vi "Init.vi"(7 "Options":T1, 8 "error in (no error)":errorcluster, 10 "Daemonized":bool, 11 "Execution in":refnum<class "Execution.lvclass">) -> (0 "error out":errorcluster, 3 "Execution out":refnum<class "Execution.lvclass">)   [LabVIEW 2020, in "TSnax.lvlib" / "Execution.lvclass"]
uses:
  Execution.lvclass
  Execution.lvclass/Execution.ctl
  Step Results.ctl
  Execution Options.ctl
  TSnax.lvlib
  Report/Report.lvclass
  SequenceFile/SequenceFile.lvclass
  PropertyObject/PropertyObject.lvclass
  Ref Data.ctl
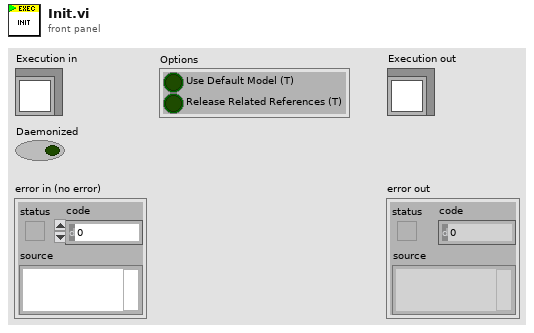
[diagram p1: front panel]
types:
  T1 = typedef "TSnax.lvlib/Execution Options.ctl" = cluster{"Use Default Model (T)":bool, "Release Related References (T)":bool}
  T2 = typedef "TSnax.lvlib/Execution.lvclass/Ref Data.ctl" = cluster{"Parameters":refnum<class "PropertyObject.lvclass">, "Client Sequence":refnum<class "SequenceFile.lvclass">, "Process Model":refnum<class "SequenceFile.lvclass">, "Entry Sequence":string, "Execution":refnum<k7>, "Report":refnum<class "Report.lvclass">, "Options":T1, "Started":bool, "Complete":bool}
  T3 = typedef "TSnax.lvlib/Execution.lvclass/Step Results.ctl" = cluster{"Map":map{string, string}}
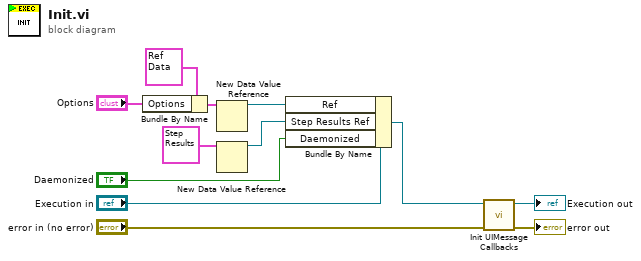
[diagram p0: block diagram]
diagram:
  n1 = Bundle By Name(cluster=T2 {"Parameters"=refnum, "Client Sequence"=refnum, "Process Model"=refnum, "Entry Sequence"="", "Execution"=refnum, "Report"=refnum, "Options"={"Use Default Model (T)"=FALSE, "Release Related References (T)"=FALSE}, "Started"=FALSE, "Complete"=FALSE} ("Ref Data"), "Options"="Options") -> (w9:T2)
  n2 = New Data Value Reference(data value=w9) -> (data value reference=w8:refnum<data-value>)  [unwired: 1 in, 1 out]
  n3 = New Data Value Reference(data value=T3 {"Map"={}} ("Step Results")) -> (data value reference=w6:refnum<data-value>)  [unwired: 1 in, 1 out]
  n4 = Bundle By Name(cluster="Execution in", "Ref"=w8, "Step Results Ref"=w6, "Daemonized"="Daemonized") -> (w3:refnum<class "Execution.lvclass">)
  n5 = call "Init UIMessage Callbacks.vi"("error in (no error)"="error in (no error)", "Execution in"=w3) -> ("error out"=→"error out":errorcluster, "Execution out"=→"Execution out":refnum<class "Execution.lvclass">)  [unwired: 8 in]
